vi "Lab3.vi"() -> ()   [LabVIEW 2019]
uses:
  <vilib>/Analysis/Matrix/Datatypes/RealMatrix.ctl
  <vilib>/Analysis/baseanly.llb/Real A x B.vi
  <vilib>/Analysis/baseanly.llb/Real Inverse Matrix.vi
  <vilib>/Analysis/NI_AALBase.lvlib
  <vilib>/Analysis/Matrix/NI_Matrix.lvlib
panel:
  out "A * B":T1
  in  "Array 2":dbl[][](array[numeric])
  in  "Array":dbl[][](array[numeric])
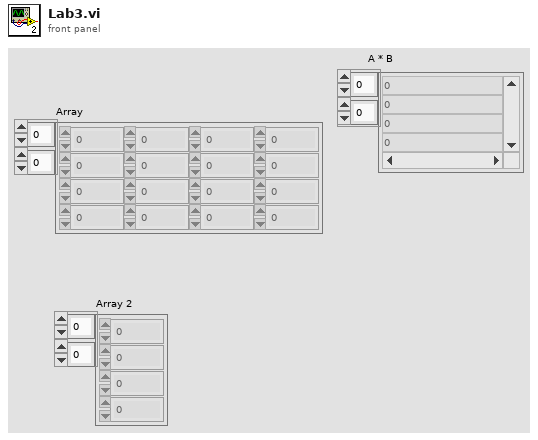
[diagram p1: front panel]
types:
  T1 = typedef "NI_Matrix.lvlib/RealMatrix.ctl" = dbl[][]
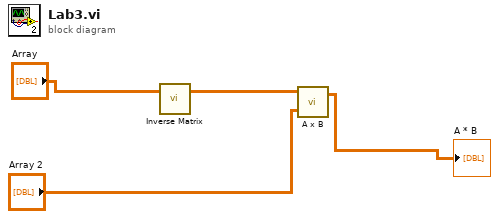
[diagram p0: block diagram]
diagram:
  n1 = call-poly <vilib>:"Inverse Matrix.vi"("Input Matrix"="Array") -> ("Inverse Matrix"=w3:T1)  [unwired: 1 in, 1 out]
  n2 = call-poly <vilib>:"A x B.vi"("B"="Array 2", "A"=w3) -> ("A x B"=→"A * B":T1)  [unwired: 1 out]
